vi "MungeInput.vi"(8 "error in (no error)":errorcluster, 10 "Input":string, 11 "UPC in":refnum<class "UPC.lvclass">) -> (0 "error out":errorcluster, 2 "Munged Input":string, 3 "UPC out":refnum<class "UPC.lvclass">)   [LabVIEW 2013, in "BarCodes.lvlib" / "UPC.lvclass"]
doc: "Modifies the input by prepending it with a 0, then calling the parent with the new input."
uses:
  UPC.lvclass
  EAN-13/EAN-13.lvclass
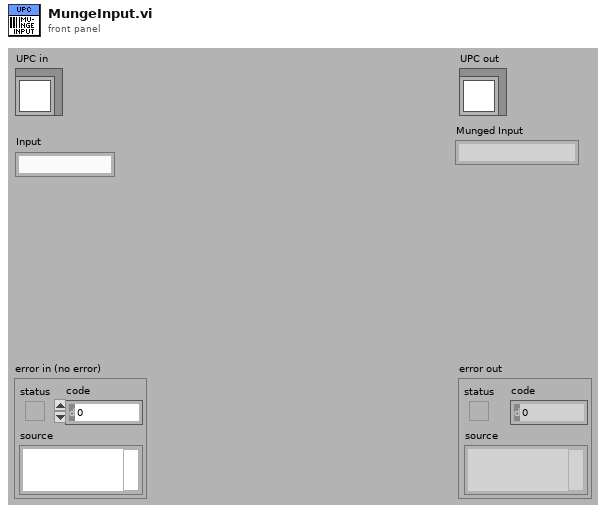
[diagram p1: front panel]
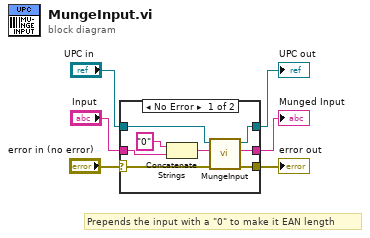
[diagram p0: block diagram]
diagram:
  # "Prepends the input with a \"0\" to make it EAN length"
  n1 = case shown="No Error" "error in (no error)" {
    selector: "error in (no error)" -> [w7 w16]
    tunnel: [w14 w15] -> w6
    tunnel: [w13 w17] -> w5
    tunnel: "UPC in" -> [w12 w17]
    tunnel: [w11 w16] -> w3
    tunnel: "Input" -> [w10 w15]
    frame No Error {
      n2 = Concatenate Strings("0" ("string"), w10) -> (w9:string)
      n3 = call-parent "MungeInput.vi"("error in (no error)"=w7, "Input"=w9, "BarCode in"=w12) -> ("error out"=w11:errorcluster, "Munged Input"=w14:string, "BarCode out"=w13:refnum<class "UPC.lvclass">)  [unwired: 6 in]
    }
    frame Error {
    }
  }
  "UPC out" <- w5
  "Munged Input" <- w6
  "error out" <- w3
